vi "dvp Vi Get Roi Descr.vi"(0 "handle":u32, 1 "piMaxH":i32, 2 "piStepH":i32, 5 "piMinW":i32, 7 "piMinH":i32, 9 "piMaxW":i32, 12 "piStepW":i32) -> (3 "piMaxH out":i32, 4 "piStepH out":i32, 6 "piMinW out":i32, 8 "piMinH out":i32, 10 "piMaxW out":i32, 13 "function return":u32(ring), 14 "piStepW out":i32)   [LabVIEW 2018, in "LabViewDVPCamera.lvlib"]
doc: "LabviewDvp2Api dvpStatus dvpViGetRoiDescr(\n dvpHandle handle, \n dvpInt32 *piMinW,\n dvpInt32 *piMinH,\n dvpInt32 *piMaxW,\n dvpInt32 *piMaxH,\n dvpInt32 *piStepW,\n dvpInt32 *piStepH);"
uses:
  LabViewDVPCamera.lvlib
  LabViewDVPCamera/LabViewDVPCamera.dll
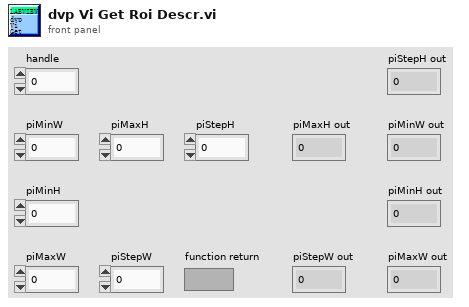
[diagram p1: front panel]
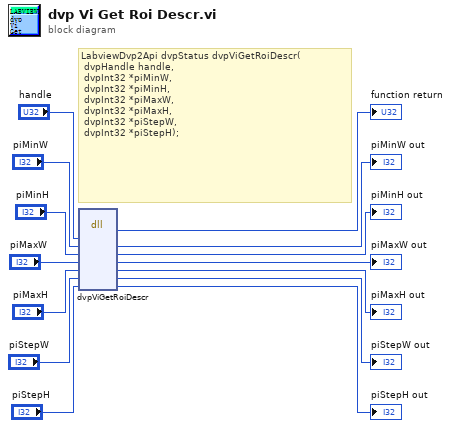
[diagram p0: block diagram]
diagram:
  # "LabviewDvp2Api dvpStatus dvpViGetRoiDescr(\n\tdvpHandle handle, \n\tdvpInt32 *piMinW,\n\tdvpInt32 *piMinH,\n\tdvpInt32 *piMaxW,\n\tdvpInt32 *piMaxH,\n\tdvpInt32 *piStepW,\n\tdvpInt32 *piStepH);"
  n1 = dll-call lib="C:/Program Files (x86)/DVP2 Labview cn 64/Sample/LabViewDVPCamera/LabViewDVPCamera.*" fn="dvpViGetRoiDescr"("handle"="handle", "piMinW"="piMinW", "piMinH"="piMinH", "piMaxW"="piMaxW", "piMaxH"="piMaxH", "piStepW"="piStepW", "piStepH"="piStepH") -> (→"function return":u32, "piMinW"=→"piMinW out":i32, "piMinH"=→"piMinH out":i32, "piMaxW"=→"piMaxW out":i32, "piMaxH"=→"piMaxH out":i32, "piStepW"=→"piStepW out":i32, "piStepH"=→"piStepH out":i32)  [unwired: 4 in, 2 out]
